vi "full command.vi"(1 "Command string":string) -> (0 "Full command":bool)   [LabVIEW 2016]
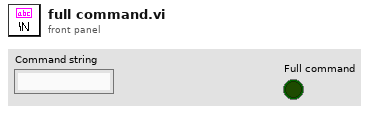
[diagram p1: front panel]
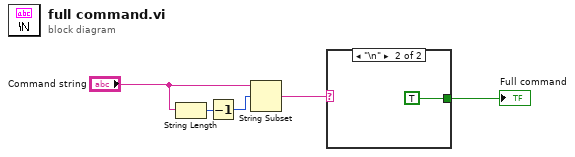
[diagram p0: block diagram]
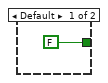
[diagram p2: hidden frame]
diagram:
  n1 = String Length(string="Command string") -> (length=w4:i32)
  n2 = Decrement(x=w4) -> (x-1=w3:i32)
  n3 = String Subset(string="Command string", offset (0)=w3) -> (substring=w1:string)  [unwired: 1 in]
  n4 = case shown="\"\\n\"" w1 {
    tunnel: [FALSE ("Full command") TRUE ("Full command")] -> w5
    frame Default {
    }
    frame "\n" {
    }
  }
  "Full command" <- w5
